vi "Helper - BuoyPoints.vi"(7 "Distance":dbl=2.0, 9 "K":dbl, 10 "East":dbl, 11 "North":dbl) -> (0 "NorthOut 2":dbl, 1 "East Out 2":dbl, 2 "NorthOut":dbl, 3 "East Out":dbl)   [LabVIEW 2011]
panel:
  # "2m distance to buoy Default Value\nCan be changed depending on Waypoint precision"
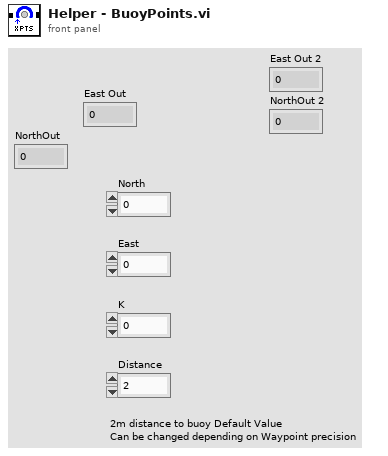
[diagram p1: front panel]
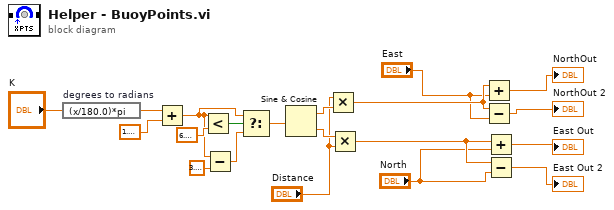
[diagram p0: block diagram]
diagram:
  n1 = expression code="(x/180.0)*pi" "degrees to radians"("K") -> (w19:dbl)
  n2 = Add(x=w19, y=1.5707963267948966) -> (x+y=w13:dbl)
  n3 = Less?(x=w13, y=6.283185307179586) -> (x < y?=w16:bool)
  n4 = Subtract(x=w13, y=3.141592653589793) -> (x-y=w14:dbl)
  n5 = Select(t=w13, s=w16, f=w14) -> (s? t:f=w12:dbl)
  n6 = Sine & Cosine(0:w12) -> (1:w11:dbl, 2:w10:dbl)
  n7 = Multiply(x="Distance", y=w11) -> (x*y=w6:dbl)
  n8 = Multiply(x=w10, y="Distance") -> (x*y=w8:dbl)
  n9 = Add(x=w6, y="East") -> (x+y=→"NorthOut":dbl)
  n10 = Subtract(x=w6, y="East") -> (x-y=→"NorthOut 2":dbl)
  n11 = Add(x=w8, y="North") -> (x+y=→"East Out":dbl)
  n12 = Subtract(x=w8, y="North") -> (x-y=→"East Out 2":dbl)
